vi "FPGA.vi"() -> ()   [LabVIEW 2023]
uses:
  <vilib>/rvi/Emulation/niFpgaGetClockAttributes.vi
  <vilib>/rvi/Emulation/niFpgaSctlEmulationGetInTimedLoop.vi
  <vilib>/rvi/Emulation/niFpgaEmulationReportErrorSimple.vi
  <vilib>/rvi/eio/common/nirviEmuTemplateMethod_errors.vi
  <vilib>/eio/utilities/niEioResolveVilibRelativePath.vi
  <vilib>/rvi/interface/RandomDataEmulation/niFpgaRandomDataHandleErrors.vi
  <vilib>/rvi/Emulation/niFpgaProcessEmulError.vi
  <vilib>/rvi/Emulation/niFpgaCriticalErrorInLSC.vi
  <vilib>/eio/EIONode/EIONode.xnode
  <vilib>/eio/EIOMethodNode/EIOMethodNode.xnode
  <vilib>/rvi/DataTransferAndStorage/Container/XNode/niFpgaContainer.xnode
  <vilib>/rvi/interface/RandomDataEmulation/nirviRandomDataFpgaReadWriteTemplate.vi
panel:
  out "Open":bool[](array[boolean])
  out "Out Of Range":bool[](array[boolean])
  in  "Capture":bool
  out "Loop Count":i32
  out "Measurements":fxp<+/-,24,-2>[](array[numeric]) format="%#_10g"
  out "Busy LED":bool
  out "Timed Out?":bool
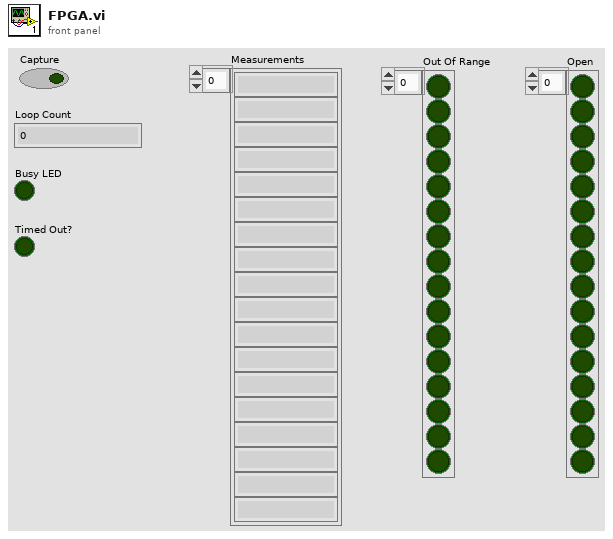
[diagram p1: front panel]
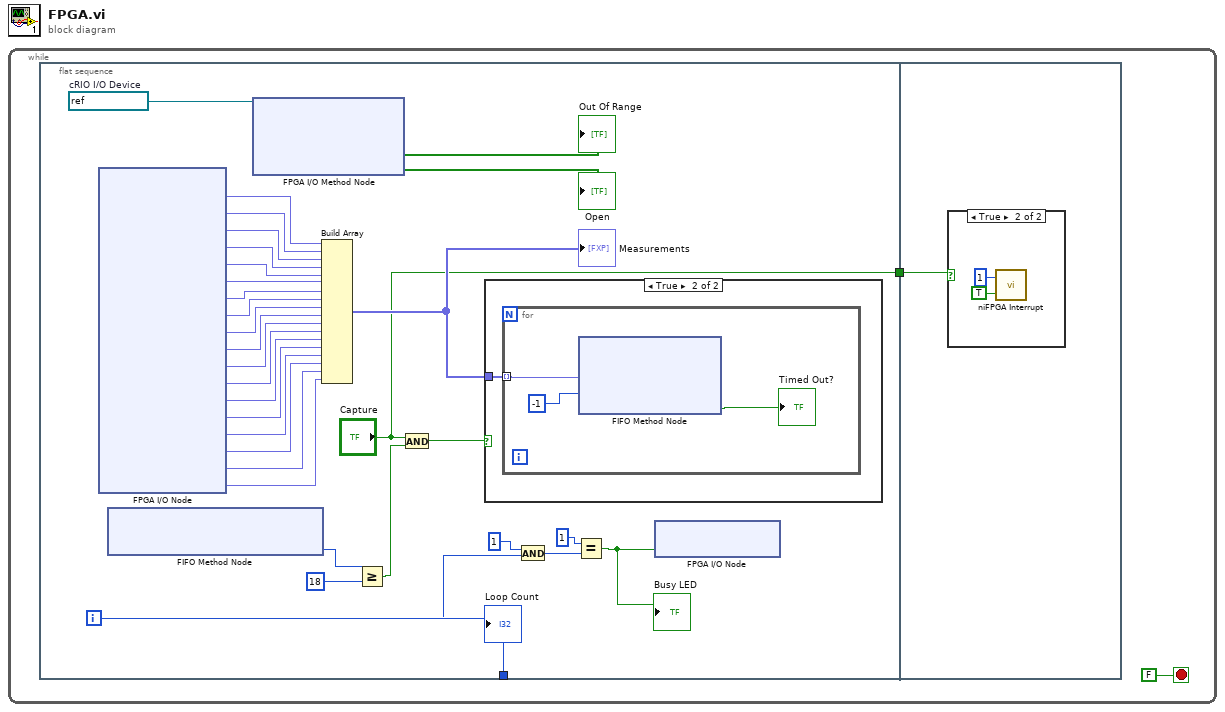
[diagram p0: block diagram]
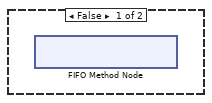
[diagram p2: hidden frame]
diagram:
  n1 = while {
    i -> [w2]
    stop <- FALSE stop-if-true
    n2 = flat-sequence {
      tunnel: w2 -> [w12]
      tunnel: ["Capture"] -> w1
      tunnel: w1 -> [w40]
      frame #0 {
        w5 = refnum<k21> "Thermal 1"  # cRIO I/O Device
        n3 = xnode "FPGA I/O Node"() -> ("TC0"=w35:fxp<+/-,24,-2>, "TC1"=w34:fxp<+/-,24,-2>, "Mod1/TC2"=w33:fxp<+/-,24,-2>, "Mod1/TC3"=w32:fxp<+/-,24,-2>, "Mod1/TC4"=w31:fxp<+/-,24,-2>, "Mod1/TC5"=w30:fxp<+/-,24,-2>, "Mod1/TC6"=w29:fxp<+/-,24,-2>, "Mod1/TC7"=w28:fxp<+/-,24,-2>, "Mod1/TC8"=w27:fxp<+/-,24,-2>, "Mod1/TC9"=w26:fxp<+/-,24,-2>, "Mod1/TC10"=w25:fxp<+/-,24,-2>, "Mod1/TC11"=w24:fxp<+/-,24,-2>, "Mod1/TC12"=w23:fxp<+/-,24,-2>, "Mod1/TC13"=w22:fxp<+/-,24,-2>, "Mod1/TC14"=w21:fxp<+/-,24,-2>, "Mod1/TC15"=w20:fxp<+/-,24,-2>, "Mod1/Autozero"=w18:fxp<+/-,24,-2>, "Mod1/CJC"=w17:fxp<+/-,24,-2>)  [unwired: 18 in, 18 out]
        n4 = xnode ("FIFO Method Node")() -> ("Number of Elements to Write"=w15:u32)  [unwired: 1 in, 1 out]
        n5 = xnode "FPGA I/O Method Node"("FPGA I/O In"=w5) -> ("Out Of Range"=→"Out Of Range":bool[], "Open"=→"Open":bool[])  [unwired: 1 in, 1 out]
        n6 = Build Array(w35, w34, w33, w32, w31, w30, w29, w28, w27, w26, w25, w24, w23, w22, w21, w20, w18, w17) -> (w19:fxp<+/-,24,-2>[])
        "Measurements" <- w19
        n7 = Greater Or Equal?(x=w15, y=u32 18) -> (x >= y?=w13:bool)
        n8 = And(x="Capture", y=w13) -> (x .and. y?=w16:bool)
        n9 = case shown="True" w16 {
          tunnel: w19 -> [_ w36]
          frame False {
            n10 = xnode ("FIFO Method Node")() -> ()  [unwired: 1 in, 1 out]
          }
          frame True {
            n11 = for {
              tunnel: w36 -> [w39] mode=indexing
              n12 = xnode ("FIFO Method Node")("Element"=w39, "Timeout"=-1) -> ("Timed Out?"=→"Timed Out?":bool)  [unwired: 1 in, 1 out]
            }
          }
        }
        n13 = And(x=1, y=w12) -> (x .and. y?=w10:i32)
        n14 = Equal?(x=1, y=w10) -> (x = y?=w8:bool)
        "Busy LED" <- w8
        n15 = xnode "FPGA I/O Node"("USER FPGA LED"=w8) -> ()  [unwired: 1 in, 1 out]
        "Loop Count" <- w12
      }
      frame #1 {
        n16 = case shown="True" w40 {
          frame False {
          }
          frame True {
            n17 = call <vilib>:"niFPGA Interrupt.vi"("Wait Until Cleared (F)"=TRUE, "IRQ Number (0)"=u8 1) -> ()  [unwired: 1 in]
          }
        }
      }
    }
  }
